vi "Meas MagField.vi"(3 "error in (no error)":errorcluster, 5 "VISA resource name":refnum<visa-resource-name>) -> (0 "error out":errorcluster, 2 "Field Level":dbl[unit])   [LabVIEW 2017]
panel:
  in  "Write/Read delay (ms)":i16
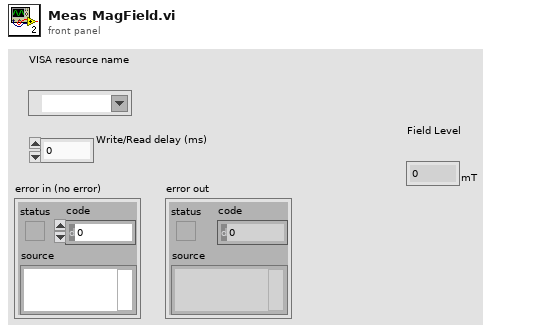
[diagram p1: front panel]
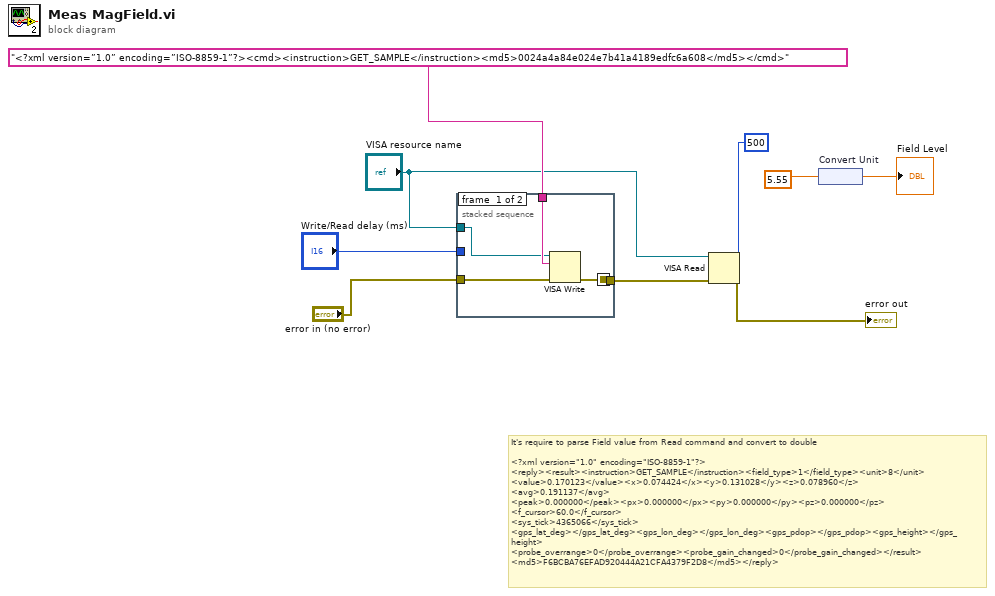
[diagram p0: block diagram]
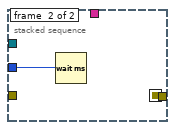
[diagram p2: hidden frame]
diagram:
  # "It's require to parse Field value from Read command and convert to double\n\n<?xml version=\"1.0\" encoding=\"ISO-8859-1\"?>\n<reply><result><instruction>GET_SAMPLE</instruction><field_type>1</field_type><unit>8</unit>\n<value>0.170123</value><x>0.074424</x><y>0.131028</y><z>0.078960</z>\n<avg>0.191137</avg>\n<peak>0.000000</peak><px>0.000000</px><py>0.000000</py><pz>0.000000</pz>\n<f_cursor>60.0</f_cursor>\n<sys_tick>4365066</sys_tick>\n<gps_lat_deg></gps_lat_deg><gps_lon_deg></gps_lon_deg><gps_pdop></gps_pdop><gps_height></gps_height>\n<probe_overrange>0</probe_overrange><probe_gain_changed>0</probe_gain_changed></result>\n<md5>F6BCBA76EFAD920444A21CFA4379F2D8</md5></reply>"
  n1 = stacked-sequence {
    seq-local: [w10 _] -> [_ w15]
    tunnel: "error in (no error)" -> [w13 _]
    tunnel: "<?xml version=”1.0” encoding=”ISO-8859-1”?><cmd><instruction>GET_SAMPLE</instruction><md5>0024a4a84e024e7b41a4189edfc6a608</md5></cmd>" -> [w12 _]
    tunnel: "VISA resource name" -> [w11 _]
    tunnel: [_ w15] -> w5
    tunnel: "Write/Read delay (ms)" -> [_ w14]
    frame #0 {
      n2 = VISA Write(VISA resource name=w11, write buffer=w12, error in (no error)=w13) -> (error out=w10:errorcluster)  [unwired: 2 out]
    }
    frame #1 {
      n3 = Wait (ms)(milliseconds to wait=w14) -> ()  [unwired: 1 out]
    }
  }
  n4 = VISA Read(VISA resource name="VISA resource name", byte count=500, error in (no error)=w5) -> (error out=→"error out":errorcluster)  [unwired: 3 out]
  n5 = node "Convert Unit"(5.55) -> (→"Field Level":dbl[unit])
